vi "Dispense FN - OFF - Measure Slope -2 (SubVI).vi"(0 "Measured Mass (g)":dbl(knob) scale=0.0..100.0, 2 "Settings":T1={"ON Settings"={"Enable Dynamic Setpoint?"=TRUE, "Enable Dynamic Dispense Time?"=TRUE, "Enable Drain Rate Functions"=TRUE, "Dispense Sample Time (s)"=0.5, "Dispense Slope Ave"=0, "ON Timeout (sec)"=600.0, "1st Setpoint (% of Target)"=0.0, "2nd Setpoint (% of Target)"=0.0, "3rd Setpoint (% of Target)"=0.0, "Measure Dispense Delay (sec)"=0.0, "Settle Slope Sample Time (s)"=0.0}, "OFF Settings"={"Drain Sample Time (s)"=0.5, "Drain Rate Ave Size"=5, "Drain Rate Limits (± g/sec)"=10.0, "Level Slope Range (± g/sec)"=0.25, "OFF Timeout (sec)"=0.0, "Near SP Slope Level (± g/sec)"=0.01, "Near Setpoint Threshold (%)"=95.0}, "Overshoot Settings"={"Time Limit (s)"=60.0, "Container MAX (g)"=1500.0, "Max FILL Slope (+/- g/sec)"=10.0, "% Overshot to Enable (>)"=0.25}, "FILL Timeout (s)"=300.0, "Full Settle Time (s)"=3.0, "Pre-Hydrate \nSpray Time (s)"=10.0, "Pre-Hydrate \nWait Time (s)"=30.0}, 3 "Static Setpoint (g)":dbl, 5 "Initialize":bool) -> (14 "Level Signal":bool, 15 "Ave. Slope (g/sec)":dbl, 16 "Rate (g/sec)":dbl, 17 "Time (s)":dbl, 18 "Level Count":i32)   [LabVIEW 2012]
uses:
  <vilib>/ptbypt/NI_PtbyPt.lvlib
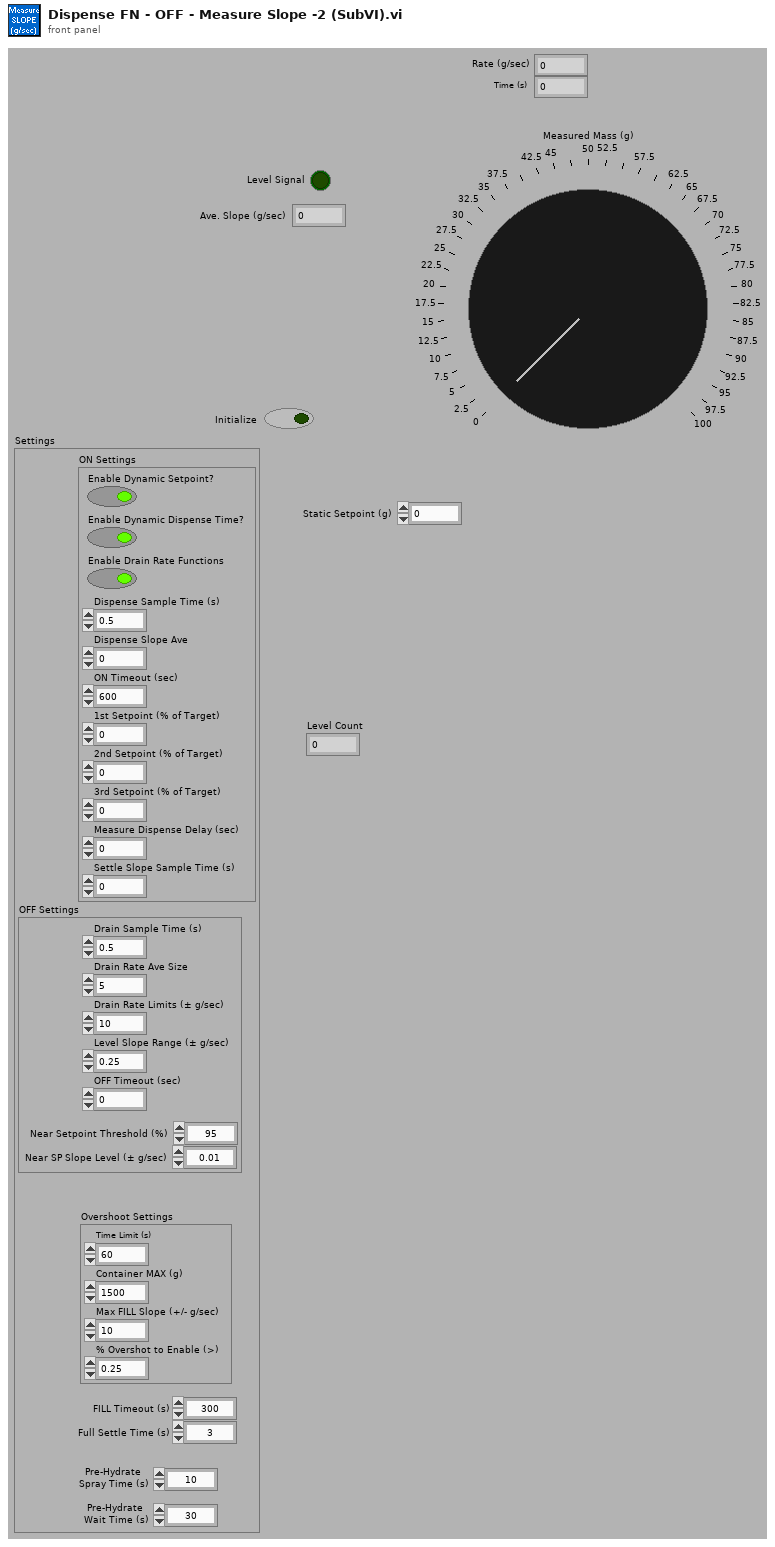
[diagram p1: front panel]
types:
  T1 = cluster{"ON Settings":cluster{"Enable Dynamic Setpoint?":bool, "Enable Dynamic Dispense Time?":bool, "Enable Drain Rate Functions":bool, "Dispense Sample Time (s)":dbl, "Dispense Slope Ave":i32, "ON Timeout (sec)":dbl, "1st Setpoint (% of Target)":dbl, "2nd Setpoint (% of Target)":dbl, "3rd Setpoint (% of Target)":dbl, "Measure Dispense Delay (sec)":dbl, "Settle Slope Sample Time (s)":dbl}, "OFF Settings":cluster{"Drain Sample Time (s)":dbl, "Drain Rate Ave Size":i32, "Drain Rate Limits (± g/sec)":dbl, "Level Slope Range (± g/sec)":dbl, "OFF Timeout (sec)":dbl, "Near SP Slope Level (± g/sec)":dbl, "Near Setpoint Threshold (%)":dbl}, "Overshoot Settings":cluster{"Time Limit (s)":dbl, "Container MAX (g)":dbl, "Max FILL Slope (+/- g/sec)":dbl, "% Overshot to Enable (>)":dbl}, "FILL Timeout (s)":dbl, "Full Settle Time (s)":dbl, "Pre-Hydrate \nSpray Time (s)":dbl, "Pre-Hydrate \nWait Time (s)":dbl}
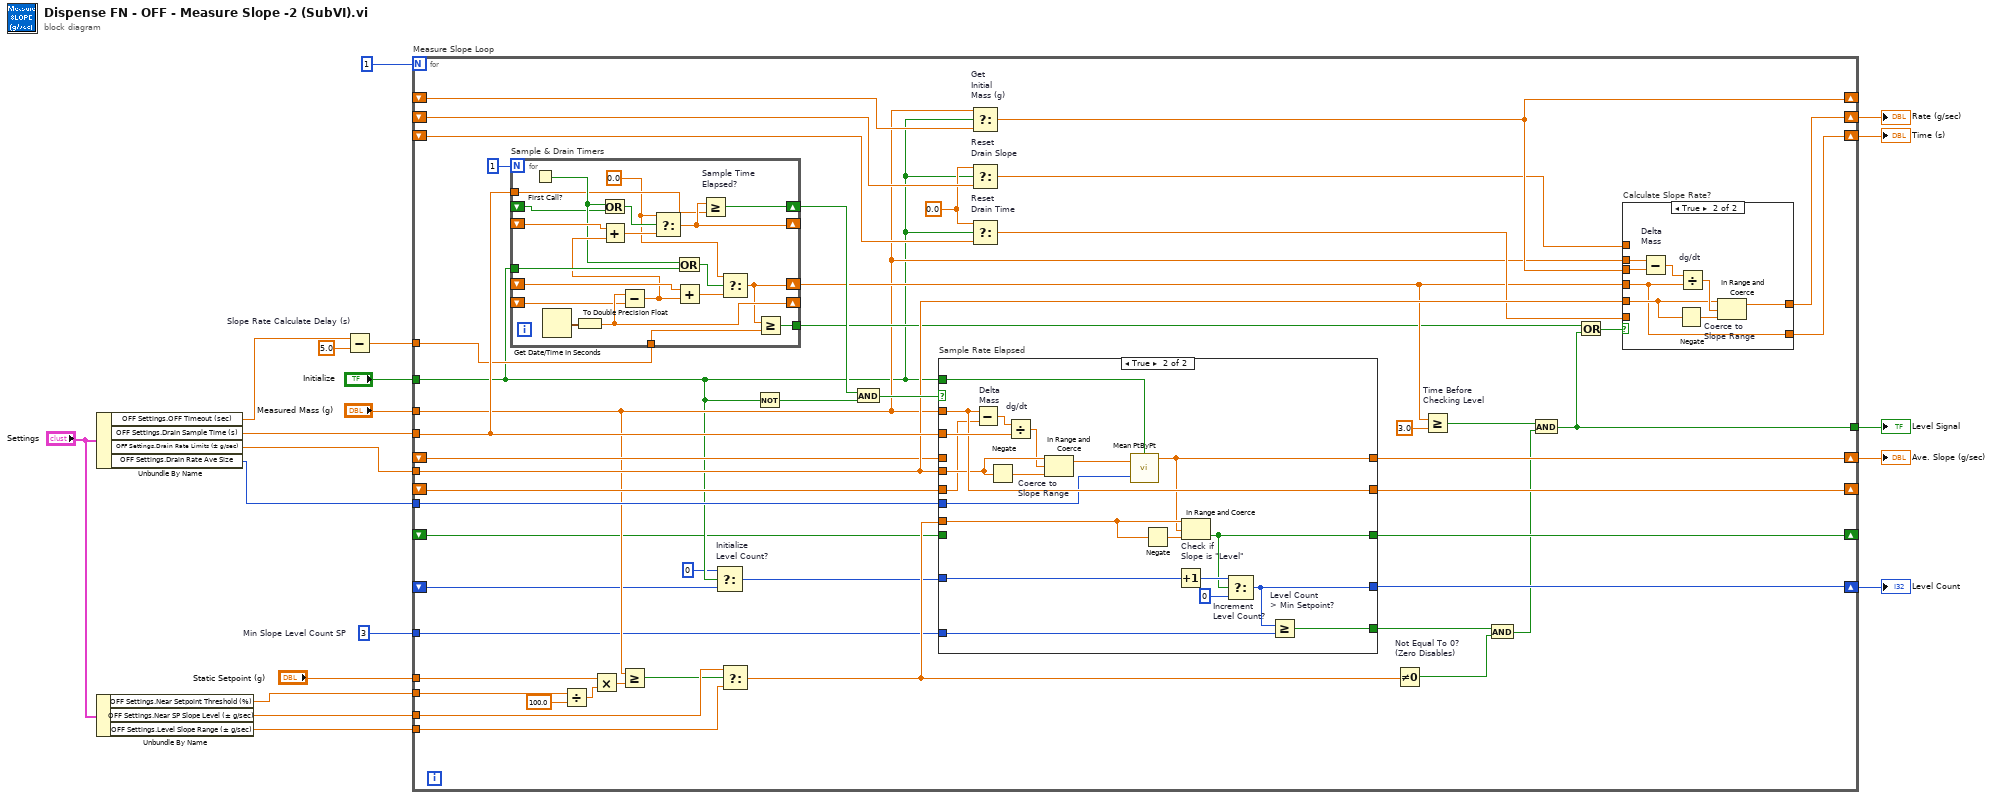
[diagram p0: block diagram]
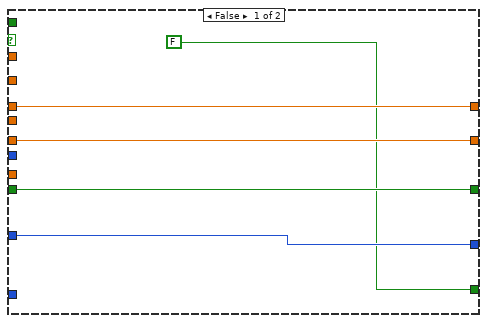
[diagram p3: hidden frame]
diagram:
  w2 = 3  # Min Slope Level Count SP
  n1 = Unbundle By Name("Settings") -> ("OFF Settings.Near Setpoint Threshold (%)"=w12:dbl, "OFF Settings.Near SP Slope Level (± g/sec)"=w11:dbl, "OFF Settings.Level Slope Range (± g/sec)"=w10:dbl)
  n2 = Unbundle By Name("Settings") -> ("OFF Settings.OFF Timeout (sec)"=w8:dbl, "OFF Settings.Drain Sample Time (s)"=w5:dbl, "OFF Settings.Drain Rate Limits (± g/sec)"=w4:dbl, "OFF Settings.Drain Rate Ave Size"=w3:i32)
  n3 = Subtract "Slope Rate Calculate Delay (s)"(x=w8, y=5.0) -> (x-y=w6:dbl)
  n4 = for "Measure Slope Loop" {
    N: 1 -> [_]
    tunnel: "Measured Mass (g)" -> [w39]
    shift-right: [w68] -> _
    shift-left: _ -> [w51]
    shift-right: [w52] -> w19
    shift-left: _ -> [w50]
    tunnel: w5 -> [w64]
    tunnel: "Initialize" -> [w33]
    tunnel: w4 -> [w60]
    tunnel: w11 -> [w38]
    tunnel: w3 -> [w66]
    shift-right: [w61] -> _
    shift-left: _ -> [w62]
    shift-right: [w59] -> w16
    shift-left: _ -> [w58]
    shift-right: [w56] -> w15
    shift-left: _ -> [w55]
    tunnel: [w22] -> w14
    tunnel: "Static Setpoint (g)" -> [w44]
    tunnel: w12 -> [w42]
    tunnel: w10 -> [w37]
    tunnel: w6 -> [w36]
    shift-right: [w34] -> w1
    shift-left: _ -> [w31]
    shift-right: [w29] -> _
    shift-left: _ -> [w28]
    tunnel: w2 -> [w27]
    w54 = 0.0 ("t")
    n5 = for "Sample & Drain Timers" {
      N: 1 -> [_]
      shift-right: [w80] -> w48
      shift-left: _ -> [w98]
      shift-right: [w94] -> _
      shift-left: _ -> [w93]
      tunnel: w33 -> [w92]
      shift-right: [w88] -> _
      shift-left: _ -> [w87]
      tunnel: w64 -> [w85]
      shift-right: [w84] -> w63
      shift-left: _ -> [w82]
      tunnel: w36 -> [w81]
      tunnel: [w79] -> w46
      w83 = 0.0 ("t")
      n6 = First Call?() -> (First Call?: T/F=w86:bool)
      n7 = Get Date/Time In Seconds() -> (seconds since 1Jan1904=w97:timestamp)
      n8 = To Double Precision Float(number=w97) -> (double precision float=w94:dbl)
      n9 = Or(x=w86, y=w82) -> (x .or. y?=w90:bool)
      n10 = Subtract(x=w94, y=w93) -> (x-y=w89:dbl)
      n11 = Add(x=w87, y=w89) -> (x+y=w91:dbl)
      n12 = Select(t=w83, s=w90, f=w91) -> (s? t:f=w88:dbl)
      n13 = Or(x=w86, y=w92) -> (x .or. y?=w95:bool)
      n14 = Add(x=w98, y=w89) -> (x+y=w96:dbl)
      n15 = Greater Or Equal? "Sample Time\nElapsed?"(x=w88, y=w85) -> (x >= y?=w84:bool)
      n16 = Select(t=w83, s=w95, f=w96) -> (s? t:f=w80:dbl)
      n17 = Greater Or Equal?(x=w80, y=w81) -> (x >= y?=w79:bool)
    }
    n18 = Divide(x=w42, y=100.0) -> (x/y=w41:dbl)
    n19 = Multiply(x=w44, y=w41) -> (x*y=w40:dbl)
    n20 = Greater Or Equal?(x=w39, y=w40) -> (x >= y?=w21:bool)
    n21 = Select "Initialize\nLevel Count?"(t=0 ("f"), s=w33, f=w31) -> (s? t:f=w30:i32)
    n22 = Select(t=w38, s=w21, f=w37) -> (s? t:f=w35:dbl)
    n23 = Not(x=w33) -> (.not. x?=w49:bool)
    n24 = And(x=w63, y=w49) -> (x .and. y?=w67:bool)
    n25 = case "Sample Rate Elapsed" shown="True" w67 {
      tunnel: w39 -> [_ w121]
      tunnel: [w103 w111] -> w52
      tunnel: [w102 w121] -> w68
      tunnel: w64 -> [_ w122]
      tunnel: w60 -> [_ w120]
      tunnel: w66 -> [_ w118]
      tunnel: w33 -> [_ w117]
      tunnel: w51 -> [w102 w116]
      tunnel: w50 -> [w103 _]
      tunnel: w35 -> [_ w112]
      tunnel: w30 -> [w101 w109]
      tunnel: [w101 w107] -> w34
      tunnel: [w100 w106] -> w29
      tunnel: [FALSE w105] -> w26
      tunnel: w28 -> [w100 _]
      tunnel: w27 -> [_ w104]
      frame False {
      }
      frame True {
        n26 = Subtract "Delta\nMass"(x=w121, y=w116) -> (x-y=w123:dbl)
        n27 = Negate(x=w120) -> (-x=w119:dbl)
        n28 = Divide "dg/dt"(x=w123, y=w122) -> (x/y=w114:dbl)
        n29 = In Range and Coerce "Coerce to\nSlope Range"(upper limit=w120, x=w114, lower limit=w119) -> (coerced(x)=w115:dbl)  [unwired: 1 out]
        n30 = call <vilib>:"Mean PtByPt.vi"("x"=w115, "sample length"=w118, "initialize"=w117) -> ("mean"=w111:dbl)  [unwired: 2 out]
        n31 = Negate(x=w112) -> (-x=w113:dbl)
        n32 = Increment(x=w109) -> (x+1=w110:i32)
        n33 = In Range and Coerce "Check if\nSlope is \"Level\""(upper limit=w112, x=w111, lower limit=w113) -> (In Range?=w106:bool)  [unwired: 1 out]
        n34 = Select "Increment\nLevel Count?"(t=w110, s=w106, f=0) -> (s? t:f=w107:i32)
        n35 = Greater Or Equal? "Level Count\n> Min Setpoint?"(x=w107, y=w104) -> (x >= y?=w105:bool)
      }
    }
    n36 = Select "Get\nInitial\nMass (g)"(t=w39, s=w33, f=w62) -> (s? t:f=w61:dbl)
    n37 = Select "Reset\nDrain Slope"(t=w54, s=w33, f=w58) -> (s? t:f=w57:dbl)
    n38 = Select "Reset\nDrain Time"(t=w54, s=w33, f=w55) -> (s? t:f=w53:dbl)
    n39 = Not Equal To 0? "Not Equal To 0?\n(Zero Disables)"(x=w35) -> (x != 0?=w25:bool)
    n40 = Greater Or Equal? "Time Before\nChecking Level"(x=w48, y=3.0) -> (x >= y?=w24:bool)
    n41 = And(x=w26, y=w25) -> (x .and. y?=w23:bool)
    n42 = And(x=w24, y=w23) -> (x .and. y?=w22:bool)
    n43 = Or(x=w46, y=w22) -> (x .or. y?=w45:bool)
    n44 = case "Calculate Slope Rate?" shown="True" w45 {
      tunnel: w39 -> [_ w76]
      tunnel: w61 -> [_ w72]
      tunnel: w48 -> [_ w71]
      tunnel: w60 -> [_ w74]
      tunnel: [w70 w73] -> w59
      tunnel: w57 -> [w70 _]
      tunnel: [w69 w71] -> w56
      tunnel: w53 -> [w69 _]
      frame False {
      }
      frame True {
        n45 = Subtract "Delta\nMass"(x=w76, y=w72) -> (x-y=w75:dbl)
        n46 = Negate(x=w74) -> (-x=w78:dbl)
        n47 = Divide "dg/dt"(x=w75, y=w71) -> (x/y=w77:dbl)
        n48 = In Range and Coerce "Coerce to\nSlope Range"(upper limit=w74, x=w77, lower limit=w78) -> (coerced(x)=w73:dbl)  [unwired: 1 out]
      }
    }
  }
  "Ave. Slope (g/sec)" <- w19
  "Level Signal" <- w14
  "Rate (g/sec)" <- w16
  "Time (s)" <- w15
  "Level Count" <- w1
